vi "Get ID.vi"(8 "error in (no error)":errorcluster, 11 "VISA resource name":refnum<visa-resource-name>) -> (0 "error out":errorcluster, 2 "read buffer":string, 3 "VISA resource name 2":refnum<visa-resource-name>)   [LabVIEW 2012, in "Universal Power Meter.lvlib" / "Universal Power Meter.lvclass"]
uses:
  Universal Power Meter.lvclass
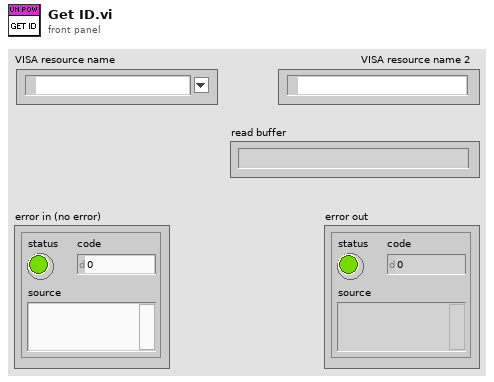
[diagram p1: front panel]
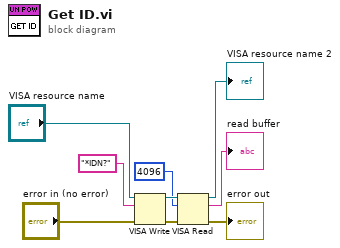
[diagram p0: block diagram]
diagram:
  n1 = VISA Write(VISA resource name="VISA resource name", write buffer="*IDN?", error in (no error)="error in (no error)") -> (VISA resource name out=w9:refnum<visa-resource-name>, error out=w8:errorcluster)  [unwired: 1 out]
  n2 = VISA Read(VISA resource name=w9, byte count=u32 4096, error in (no error)=w8) -> (VISA resource name out=→"VISA resource name 2":refnum<visa-resource-name>, read buffer=→"read buffer":string, error out=→"error out":errorcluster)  [unwired: 1 out]
